vi "DSP_SetWindowFunction.vi"(2 "error in (no error)":errorcluster, 3 "Samples Per Record":u32, 4 "Window Type":u32(ring) items=["FFT_WINDOW_NONE", "FFT_WINDOW_HANNING", "FFT_WINDOW_HAMMING", "FFT_WINDOW_BLACKMAN", "FFT_WINDOW_BLACKMAN_HARRIS", "FFT_WINDOW_BARTLETT"], 5 "Board Handle":u64) -> (0 "error out":errorcluster, 1 "Board Handle Out":u64)   [LabVIEW 2009]
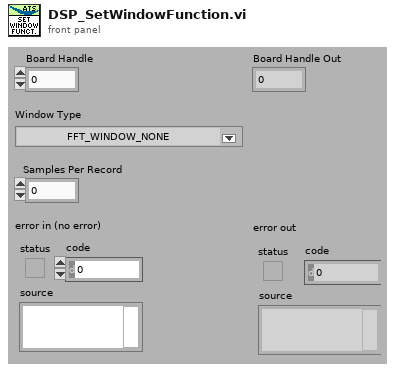
[diagram p1: front panel]
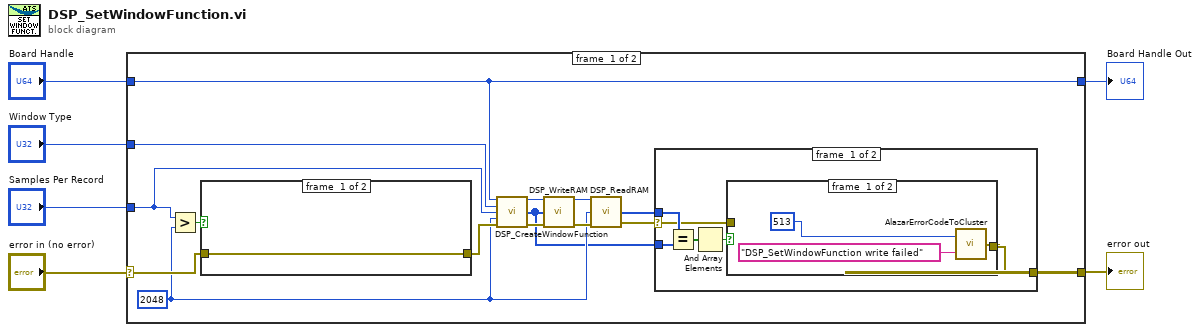
[diagram p0: block diagram]
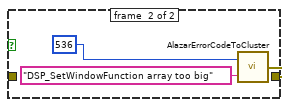
[diagram p4: hidden frame]
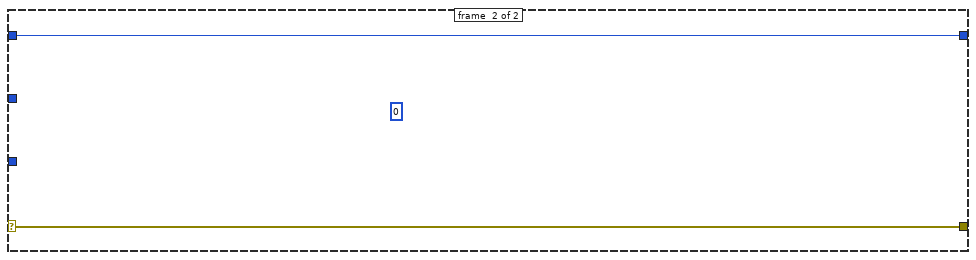
[diagram p5: hidden frame]
diagram:
  n1 = case shown="No Error" "error in (no error)" {
    selector: "error in (no error)" -> [w16 w38]
    tunnel: [w8 w38] -> w5
    tunnel: [w19 w37] -> w4
    tunnel: "Board Handle" -> [w19 w37]
    tunnel: "Samples Per Record" -> [w18 _]
    tunnel: "Window Type" -> [w20 _]
    frame #0 {
      w12 = u32 2048
      n2 = Greater?(x=w18, y=w12) -> (0:w21:bool)
      n3 = case shown="True" w21 {
        tunnel: [w33 w34] -> w17
        tunnel: w16 -> [w33 _]
        frame #0 {
        }
        frame #1 {
          n4 = call "AlazarErrorCodeToCluster.vi"("Message"="DSP_SetWindowFunction array too big", "Error Code"=u32 536) -> ("error out"=w34:errorcluster)
        }
      }
      n5 = call "DSP_CreateWindowFunction.vi"("Board Handle"=w19, "Window Type"=w20, "Samples Per Record"=w18, "Max Samples Per Record"=w12, "error in (no error)"=w17) -> ("Board Handle Out"=w14:u64, "values out"=w9:u16[], "error out"=w15:errorcluster)  [unwired: 8 in]
      n6 = call "DSP_WriteRAM.vi"("error in (no error)"=w15, "values"=w9, "Board Handle"=w14) -> ("error out"=w13:errorcluster, "Board Handle Out"=w11:u64)
      n7 = call "DSP_ReadRAM.vi"("error in (no error)"=w13, "Samples To Read"=w12, "Board Handle"=w11) -> ("error out"=w7:errorcluster, "Values Out"=w10:u16[])  [unwired: 1 out]
      n8 = case shown="No Error" w7 {
        selector: w7 -> [w23 w32]
        tunnel: w10 -> [w27 _]
        tunnel: w9 -> [w26 _]
        tunnel: [w22 w32] -> w8
        frame #0 {
          n9 = Equal?(x=w27, y=w26) -> (x = y?=w25:bool[])
          n10 = And Array Elements(Boolean array=w25) -> (logical AND=w24:bool)
          n11 = case shown="False" w24 {
            tunnel: [w28 w31] -> w22
            tunnel: w23 -> [_ w31]
            frame #0 {
              n12 = call "AlazarErrorCodeToCluster.vi"("Message"="DSP_SetWindowFunction write failed", "Error Code"=u32 513) -> ("error out"=w28:errorcluster)
            }
            frame #1 {
            }
          }
        }
        frame #1 {
        }
      }
    }
    frame #1 {
      (unwired) u32 0
    }
  }
  "Board Handle Out" <- w4
  "error out" <- w5
